vi "Get Name.vi"(11 "CD Template":refnum<class "NIVS_Timing and Sync (Abstract).lvclass">) -> (2 "String":string)   [LabVIEW 2017, in "NIVS_Timing and Sync (Abstract).lvclass"]
uses:
  NIVS_Timing and Sync (Abstract).lvclass
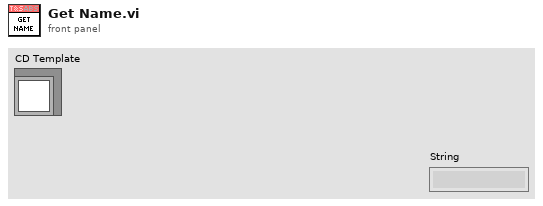
[diagram p1: front panel]
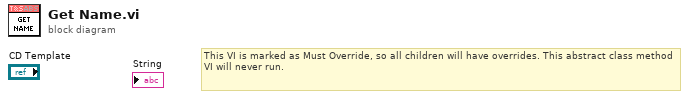
[diagram p0: block diagram]
diagram:
  # "This VI is marked as Must Override, so all children will have overrides. This abstract class method VI will never run."
